vi "execution class name.vi"(8 "error in":errorcluster, 11 "alarms module configuration in":refnum<class "alarms module configuration.lvclass">) -> (0 "error out":errorcluster, 2 "class name":string, 3 "alarms module configuration out":refnum<class "alarms module configuration.lvclass">)   [LabVIEW 2014, in "alarms module configuration.lvclass"]
doc: "Provides an interface for determining the module runtime class associated with this module configuration. This class name can then be used to dynamically load or locate the runtime class for initialization purposes."
uses:
  alarms module configuration.lvclass
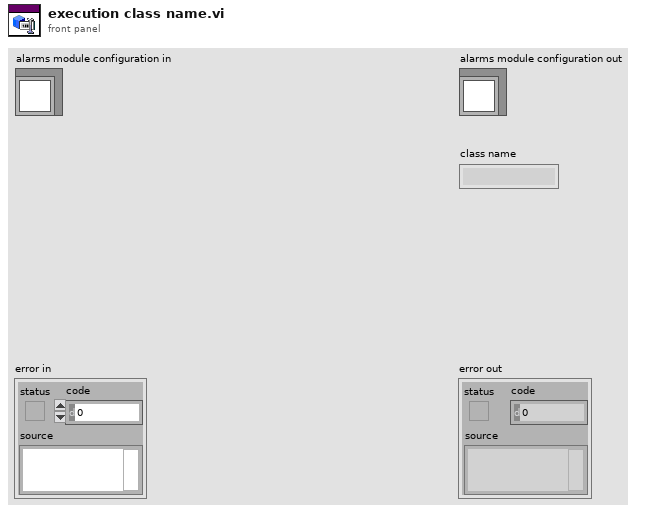
[diagram p1: front panel]
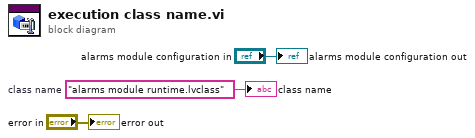
[diagram p0: block diagram]
diagram:
  w1 = "alarms module runtime.lvclass"  # class name
  "error out" <- "error in"
  "alarms module configuration out" <- "alarms module configuration in"
  "class name" <- w1
